vi "Analog Wfm Freq and Pk-Pk.vi"(10 "Channel":i32=1 min=1, 11 "Waveform Array":waveform(dbl)[](array[waveform])) -> (1 "detected frequency":dbl format="%.2p", 2 "Peak to Peak":dbl)   [LabVIEW 2010]
uses:
  <vilib>/measure/matone.llb/Extract Single Tone Information 1 Chan.vi
  <vilib>/measure/NI_MAPro.lvlib
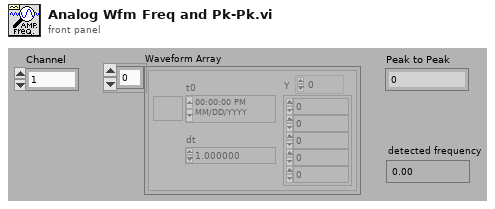
[diagram p1: front panel]
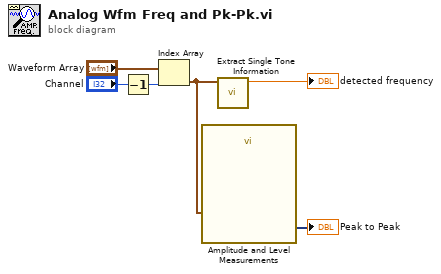
[diagram p0: block diagram]
diagram:
  n1 = Decrement(x="Channel") -> (x-1=w1:i32)
  n2 = Index Array(array="Waveform Array", index=w1) -> (element=w4:waveform(dbl))
  n3 = call "Amplitude and Level Measurements"("Signals"=w4) -> ("Peak to Peak"=→"Peak to Peak":dynamicdata)  [unwired: 13 in, 1 out]
  n4 = call-poly <vilib>:"Extract Single Tone Information.vi"("time signal in"=w4) -> ("detected frequency"=→"detected frequency":dbl)  [unwired: 5 in, 5 out]
